vi "RT_Aerodynamic_Force_in_DLR_Navigation_Reference_System (SubVI).vi"(0 "Data":dbl[][](array[numeric]), 1 "AoA_pitch (rad)":dbl, 2 "AoA_yaw (rad)":dbl, 5 "i":i32, 9 "DCM":dbl[][](array[numeric]), 11 "Sref [m^2]":dbl, 13 "Pdin":dbl) -> (4 "FA":dbl[](array[numeric]))   [LabVIEW 2017]
uses:
  <vilib>/Analysis/coordinate.llb/Euler Rotation Order.ctl
  <vilib>/Analysis/NI_AALPro.lvlib
panel:
  out "FAl":dbl[](array[numeric])
  out "FAy":dbl[](array[numeric])
  out "FAp":dbl[](array[numeric])
  out "FA_long":dbl
  out "FA_yaw":dbl
  out "FA_pitch":dbl
  out "Sref - Area de referencia":dbl=1.72 format="%#_13g"
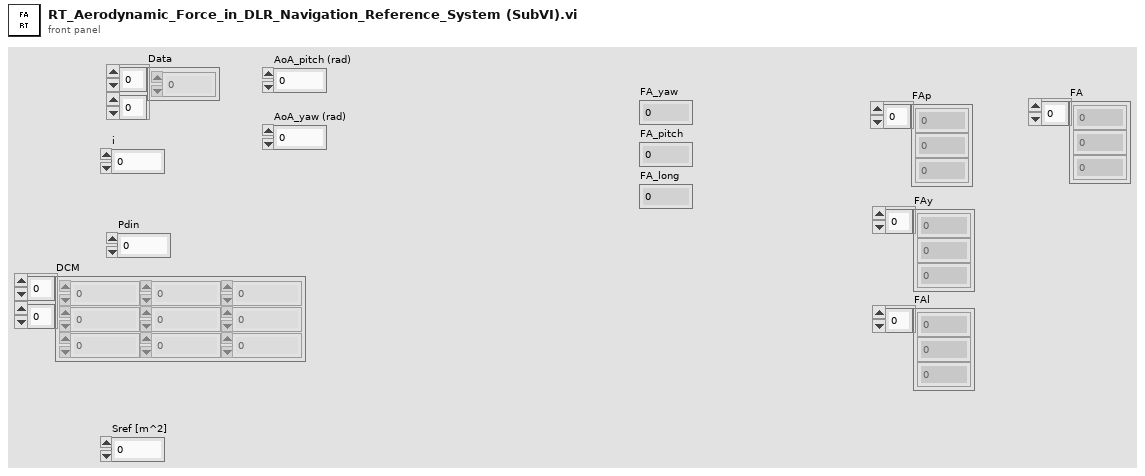
[diagram p1: front panel]
types:
  T1 = typedef "NI_AALPro.lvlib/Euler Rotation Order.ctl" = u16
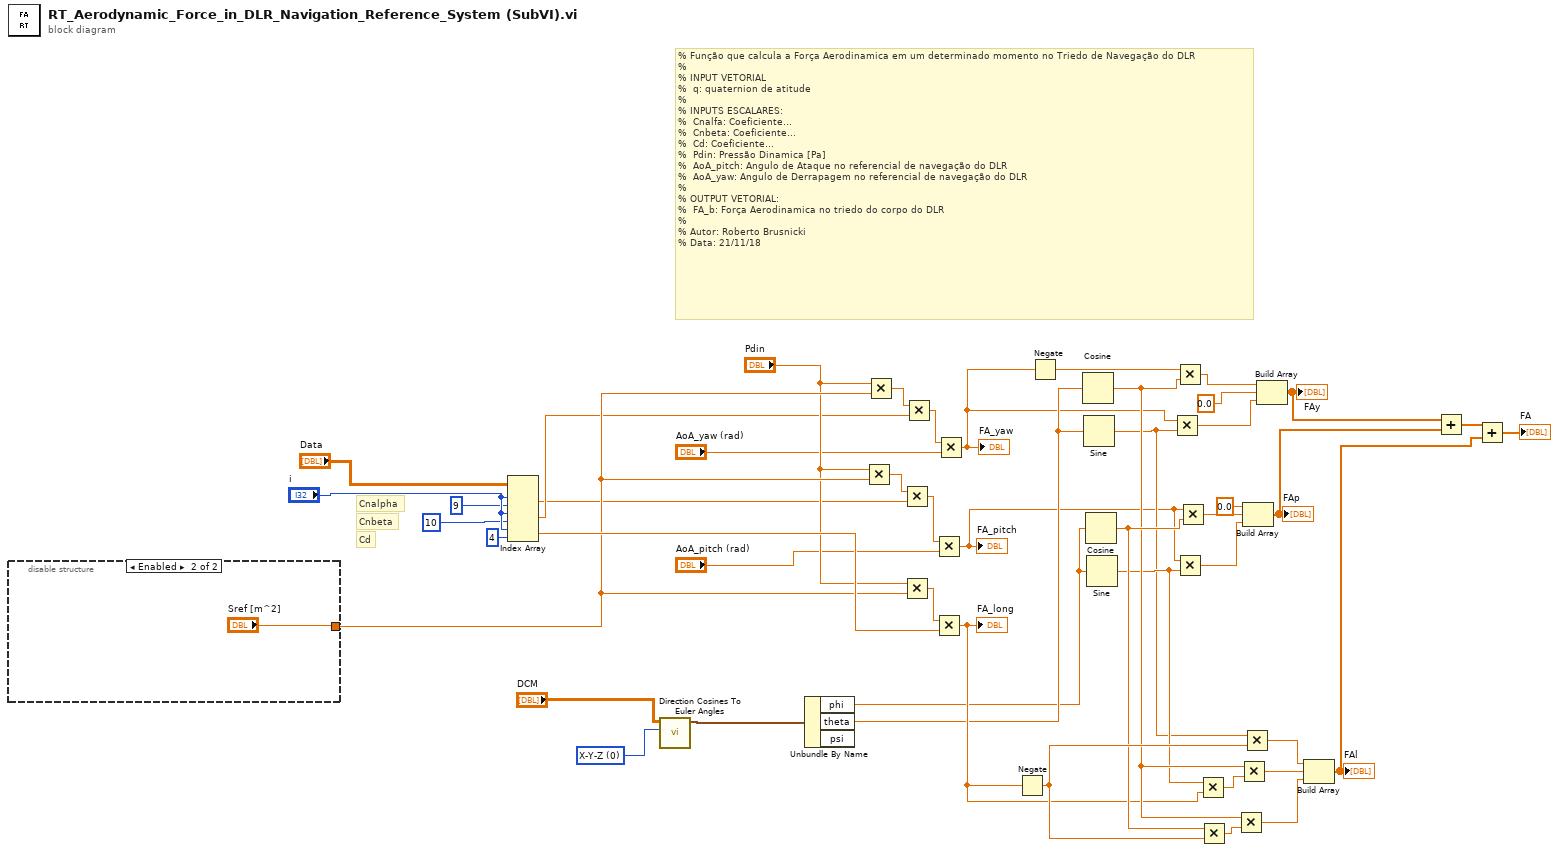
[diagram p0: block diagram]
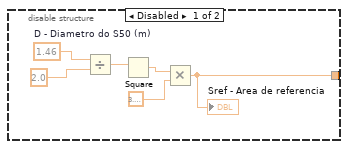
[diagram p2: hidden frame]
diagram:
  w7 = T1 0 items=["X-Y-Z", "X-Z-Y", "Y-X-Z", "Y-Z-X", "Z-X-Y", "Z-Y-X", "X-Y-X", "X-Z-X", "Y-X-Y", "Y-Z-Y", "Z-X-Z", "Z-Y-Z"] ("rotation order")
  # "% Função que calcula a Força Aerodinamica em um determinado momento no Triedo de Navegação do DLR\n%\n% INPUT VETORIAL\n%  q: quaternion de atitude\n%\n% INPUTS ESCALARES:\n%  Cnalfa: Coeficiente...\n%  Cnbeta: Coeficiente...\n%  Cd: Coeficiente...\n%  Pdin: Pressão Dinamica [Pa]\n%  AoA_pitch: Angulo de Ataque no referencial de navegação do DLR\n%  AoA_yaw: Angulo de Derrapagem no referencial de navegação do DLR\n%\n% OUTPUT VETORIAL:\n%  FA_b: Força Aerodinamica no triedo do corpo do DLR\n%\n% Autor: Roberto Brusnicki\n% Data: 21/11/18"
  # "Cd"
  # "Cnbeta"
  # "Cnalpha"
  n1 = disable-structure shown="Enabled" {
    disable-tunnel: [w53 "Sref [m^2]"] -> w18
    frame Disabled {
      w48 = 1.46  # D - Diametro do S50 (m)
      n2 = Divide(x=w48, y=2.0) -> (x/y=w51:dbl)
      n3 = Square(x=w51) -> (x^2=w52:dbl)
      n4 = Multiply(x=w52, y=3.141592653589793) -> (x*y=w53:dbl)
      "Sref - Area de referencia" <- w53
    }
    frame Enabled {
    }
  }
  n5 = Index Array(array="Data", index (row) #1="i", index (col) #1=9 ("disabled index (col)"), index (row) #2="i", index (col) #2=10 ("disabled index (col)"), index (row) #3="i", index (col) #3=4 ("disabled index (col)")) -> (element #1=w8:dbl, element #2=w14:dbl, element #3=w19:dbl)
  n6 = call <vilib>:"Direction Cosines To Euler Angles.vi"("rotation order"=w7, "Direction Cosines"="DCM") -> ("Euler Angles"=w20:cluster{"phi":dbl, "theta":dbl, "psi":dbl})  [unwired: 8 in, 1 out]
  n7 = Unbundle By Name(w20) -> ("phi"=w22:dbl, "theta"=w28:dbl)  [unwired: 1 out]
  n8 = Multiply(x="Pdin", y=w18) -> (x*y=w9:dbl)
  n9 = Multiply(x="Pdin", y=w18) -> (x*y=w13:dbl)
  n10 = Multiply(x=w9, y=w8) -> (x*y=w11:dbl)
  n11 = Multiply(x="Pdin", y=w18) -> (x*y=w16:dbl)
  n12 = Multiply(x=w13, y=w14) -> (x*y=w12:dbl)
  n13 = Multiply(x=w11, y="AoA_pitch (rad)") -> (x*y=w21:dbl)
  "FA_pitch" <- w21
  n14 = Multiply(x=w16, y=w19) -> (x*y=w38:dbl)
  "FA_long" <- w38
  n15 = Multiply(x=w12, y="AoA_yaw (rad)") -> (x*y=w26:dbl)
  "FA_yaw" <- w26
  n16 = Negate(x=w38) -> (-x=w42:dbl)
  n17 = Negate(x=w26) -> (-x=w27:dbl)
  n18 = Cosine(x=w28) -> (cos(x)=w39:dbl)
  n19 = Sine(x=w28) -> (sin(x)=w35:dbl)
  n20 = Cosine(x=w22) -> (cos(x)=w41:dbl)
  n21 = Sine(x=w22) -> (sin(x)=w37:dbl)
  n22 = Multiply(x=w26, y=w35) -> (x*y=w30:dbl)
  n23 = Multiply(x=w27, y=w39) -> (x*y=w29:dbl)
  n24 = Multiply(x=w21, y=w37) -> (x*y=w23:dbl)
  n25 = Multiply(x=w21, y=w41) -> (x*y=w24:dbl)
  n26 = Multiply(x=w37, y=w38) -> (x*y=w36:dbl)
  n27 = Multiply(x=w41, y=w42) -> (x*y=w40:dbl)
  n28 = Multiply(x=w39, y=w40) -> (x*y=w32:dbl)
  n29 = Multiply(x=w39, y=w36) -> (x*y=w33:dbl)
  n30 = Multiply(x=w35, y=w42) -> (x*y=w34:dbl)
  n31 = Build Array(0.0 ("element"), w24, w23) -> (w44:dbl[])
  "FAp" <- w44
  n32 = Build Array(w29, 0.0 ("element"), w30) -> (w43:dbl[])
  "FAy" <- w43
  n33 = Build Array(w34, w33, w32) -> (w46:dbl[])
  "FAl" <- w46
  n34 = Add(x=w43, y=w44) -> (x+y=w45:dbl[])
  n35 = Add(x=w45, y=w46) -> (x+y=→"FA":dbl[])
